vi "UT - Get Fields.vi"() -> (0 "error out":errorcluster, 2 "Fieldnames":string[](array[string]), 3 "Array":i32[](array[numeric]))   [LabVIEW 2019, in "HDF5 Tools.lvlib"]
uses:
  HDF5 Tools.lvlib
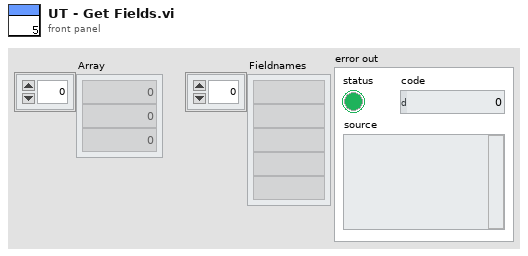
[diagram p1: front panel]
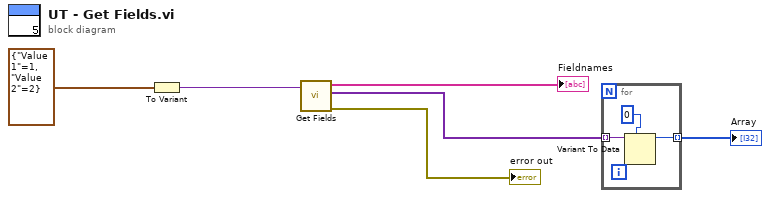
[diagram p0: block diagram]
diagram:
  n1 = To Variant(anything=cluster{"Value 1":i32, "Value 2":i32} {"Value 1"=1, "Value 2"=2}) -> (Variant=w5:variant)
  n2 = call "Get Fields.vi"("variant"=w5) -> ("error out"=→"error out":errorcluster, "element variant array"=w2:variant[], "Fieldnames"=→"Fieldnames":string[])  [unwired: 6 in, 2 out]
  n3 = for {
    tunnel: w2 -> [w9] mode=indexing
    tunnel: [w7] -> w1 mode=indexing
    n4 = Variant To Data(type=0, Variant=w9) -> (data=w7:i32)  [unwired: 1 in, 1 out]
  }
  "Array" <- w1
